vi "Ext.vi"(8 "error in (no error)":errorcluster, 9 "Val":variant, 10 "Tag":u16, 11 "Sine in":refnum<class "Rigol DG822 Sine.lvclass">) -> (0 "error out":errorcluster, 1 "Parsed":variant, 3 "Sine out":refnum<class "Rigol DG822 Sine.lvclass">)   [LabVIEW 2021, in "Rigol DG822 UI.lvlib" / "Rigol DG822 Sine.lvlib" / "Rigol DG822 Sine.lvclass"]
uses:
  Rigol DG822 Sine.lvclass
  Rigol DG822 UI/lib/controls.llb/WaveformExtCall.ctl
  Rigol DG822 Sine.lvclass/Rigol DG822 Sine.ctl
  Rigol DG822 UI/lib/controls.llb/AllWaveformDataCluster.ctl
  Rigol DG822 UI/lib/controls.llb/DataCluster.ctl
  Rigol DG822 UI/lib/controls.llb/FT Controls Cluster.ctl
  Rigol DG822 UI/lib/controls.llb/String Indicators Cluster.ctl
  General/Files/lvlibp/Actors.lvlibp/Actors/Actors/Actors.lvclass
  D:/LabVIEW/General/Files/lvlibp/Actors.lvlibp/Actors/Actors/Actors.lvclass
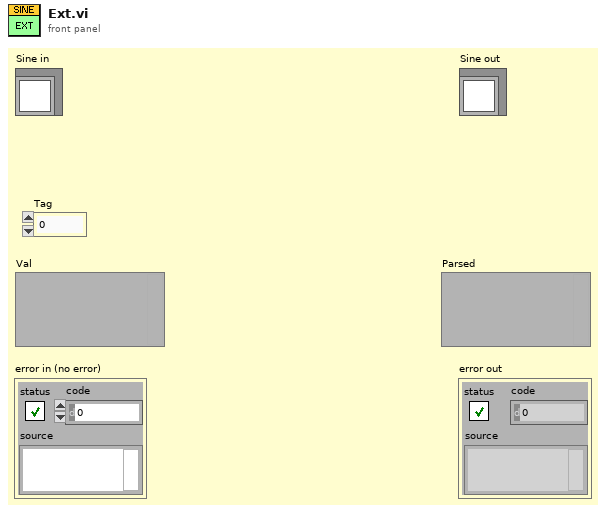
[diagram p1: front panel]
types:
  T1 = typedef "WaveformExtCall.ctl" = enum16{"Freq", "Period", "Ampl", "HighL", "Offset", "LowL", "Phase", "Duty", "Width", "RisEdge", "FallEdge", "Home", "InitData"}
  T2 = typedef "AllWaveformDataCluster.ctl" = cluster{"Data":T3, "F/T Ctrls":T4, "String Indcs":T5}
  T3 = typedef "DataCluster.ctl" = cluster{"Freq":cluster{"Freq":dbl, "FreqUnit":enum32{"No Selection", "MHz", "kHz", "Hz", "mHz", "uHz"}, "FreqUnitPrcs":dbl}, "Period":cluster{"Period":dbl, "PeriodUnit":enum32{"No Selection", "s", "ms", "us", "ns"}, "PeriodUnitPrcs":dbl}, "Ampl":cluster{"Ampl":dbl, "AmplUnit":enum32{"No Selection", "Vpp", "mVpp"}, "AmplUnitPrcs":dbl}, "HighL":cluster{"HighL":dbl, "HighLUnit":enum32{"No Selection", "V", "mV"}, "HighLUnitPrcs":dbl}, "Offset":cluster{"Offset":dbl, "OffsetUnit":enum32{"No Selection", "Vdc", "mVdc"}, "OffsetUnitPrcs":dbl}, "LowL":cluster{"LowL":dbl, "LowLUnit":enum32{"No Selection", "V", "mV"}, "LowLUnitPrcs":dbl}, "Phase":cluster{"Phase":dbl, "PhaseUnit":enum32{"°"}, "PhaseUnitPrcs":dbl}, "Duty":cluster{"Duty":dbl, "DutyUnit":enum32{"%"}, "DutyUnitPrcs":dbl}, "Width":cluster{"Width":dbl, "WidthUnit":enum32{"No Selection", "s", "ms", "us", "ns"}, "WidthUnitPrcs":dbl}, "RisEdge":cluster{"RisEdge":dbl, "RisEdgeUnit":enum32{"No Selection", "s", "ms", "us", "ns"}, "RisEdgeUnitPrcs":dbl}, "FallEdge":cluster{"FallEdge":dbl, "FallEdgeUnit":enum32{"No Selection", "s", "ms", "us", "ns"}, "FallEdgeUnitPrcs":dbl}}
  T4 = typedef "FT Controls Cluster.ctl" = cluster{"Freq/Period":bool, "Ampl/HighL":bool, "Offset/LowL":bool, "Duty/Width":bool}
  T5 = typedef "String Indicators Cluster.ctl" = cluster{"Freq-Period":string, "Ampl-HighL":string, "Offset-LowL":string, "Phase":string, "Duty-Width":string, "RisEdge":string, "FallEdge":string}
  T6 = cluster{"Freq":dbl, "FreqUnit":enum32{"No Selection", "MHz", "kHz", "Hz", "mHz", "uHz"}, "FreqUnitPrcs":dbl}
  T7 = cluster{"Period":dbl, "PeriodUnit":enum32{"No Selection", "s", "ms", "us", "ns"}, "PeriodUnitPrcs":dbl}
  T8 = cluster{"Freq":cluster{"Freq":dbl, "FreqUnit":enum32{"No Selection", "MHz", "kHz", "Hz", "mHz", "uHz"}, "FreqUnitPrcs":dbl}, "Period":cluster{"Period":dbl, "PeriodUnit":enum32{"No Selection", "s", "ms", "us", "ns"}, "PeriodUnitPrcs":dbl}}
  T9 = cluster{"Ampl":dbl, "AmplUnit":enum32{"No Selection", "Vpp", "mVpp"}, "AmplUnitPrcs":dbl}
  T10 = cluster{"HighL":dbl, "HighLUnit":enum32{"No Selection", "V", "mV"}, "HighLUnitPrcs":dbl}
  T11 = cluster{"Offset":dbl, "OffsetUnit":enum32{"No Selection", "Vdc", "mVdc"}, "OffsetUnitPrcs":dbl}
  T12 = cluster{"LowL":dbl, "LowLUnit":enum32{"No Selection", "V", "mV"}, "LowLUnitPrcs":dbl}
  T13 = cluster{"Ampl":cluster{"Ampl":dbl, "AmplUnit":enum32{"No Selection", "Vpp", "mVpp"}, "AmplUnitPrcs":dbl}, "HighL":cluster{"HighL":dbl, "HighLUnit":enum32{"No Selection", "V", "mV"}, "HighLUnitPrcs":dbl}, "Offset":cluster{"Offset":dbl, "OffsetUnit":enum32{"No Selection", "Vdc", "mVdc"}, "OffsetUnitPrcs":dbl}, "LowL":cluster{"LowL":dbl, "LowLUnit":enum32{"No Selection", "V", "mV"}, "LowLUnitPrcs":dbl}}
  T14 = cluster{"Phase":dbl, "PhaseUnit":enum32{"°"}, "PhaseUnitPrcs":dbl}
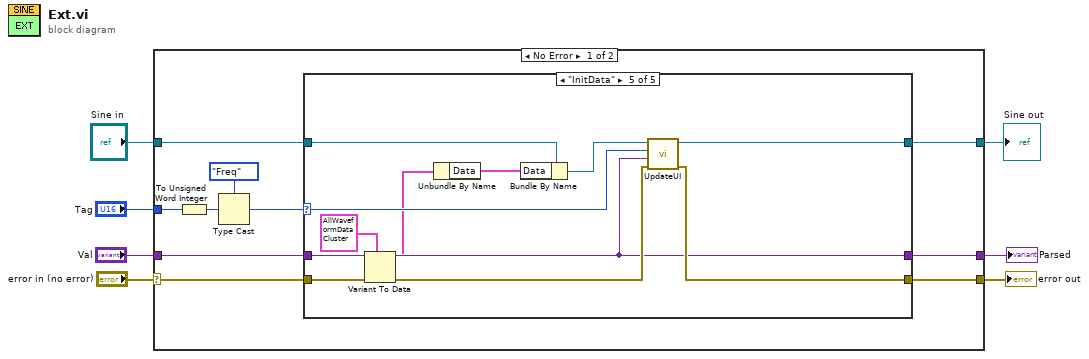
[diagram p0: block diagram]
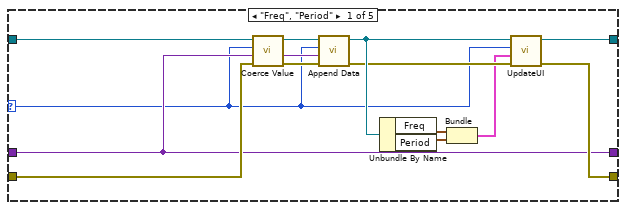
[diagram p2: hidden frame]
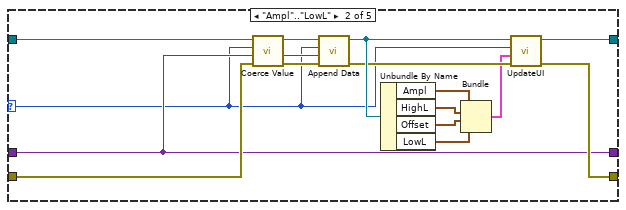
[diagram p3: hidden frame]
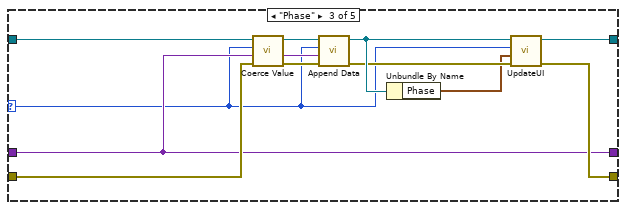
[diagram p4: hidden frame]
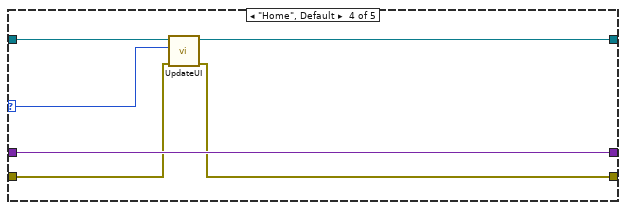
[diagram p5: hidden frame]
diagram:
  n1 = case shown="No Error" "error in (no error)" {
    selector: "error in (no error)" -> [w10 w78]
    tunnel: [w12 w77] -> w3
    tunnel: "Sine in" -> [w13 w77]
    tunnel: "Tag" -> [w16 _]
    tunnel: "Val" -> [w15 _]
    tunnel: [w11 _] -> w2
    tunnel: [w9 w78] -> w1
    frame No Error {
      n2 = To Unsigned Word Integer(number=w16) -> (unsigned 16bit integer=w17:u16)
      n3 = Type Cast(type=WaveformExtCall."Freq" ("Enum"), x=w17) -> (*(type *) &x=w14:T1)
      n4 = case shown="\"InitData\"" w14 {
        selector: w14 -> [w21 w37 w49 w63 w69]
        tunnel: w15 -> [w25 w41 w53 w62 w68]
        tunnel: w13 -> [w27 w43 w55 w65 w75]
        tunnel: [w31 w47 w59 w64 w76] -> w12
        tunnel: [w25 w41 w53 w62 w68] -> w11
        tunnel: w10 -> [w26 w42 w54 w61 w73]
        tunnel: [w30 w46 w58 w60 w70] -> w9
        frame "Freq", "Period" {
          n5 = call-dynamic "Coerce Value.vi"("error in (no error)"=w26, "Value"=w25, "ParamTags"=w21, "Rigol DG822 Sine in"=w27) -> ("error out"=w23:errorcluster, "Coerced Value"=w24:variant, "Rigol DG822 Sine out"=w28:refnum<class "Rigol DG822 Sine.lvclass">)  [unwired: 5 in]
          n6 = call-dynamic "Append Data.vi"("error in (no error)"=w23, "Data"=w24, "ParamTags"=w21, "Rigol DG822 Sine in"=w28) -> ("error out"=w22:errorcluster, "Rigol DG822 Sine out"=w29:refnum<class "Rigol DG822 Sine.lvclass">)  [unwired: 6 in]
          n7 = Unbundle By Name(w29) -> ("Freq"=w19:T6, "Period"=w18:T7)
          n8 = Bundle("Freq"=w19, "Period"=w18) -> (w20:T8)  [unwired: 1 in]
          n9 = call "UpdateUI.vi"("error in (no error)"=w22, "Data"=w20, "Type"=w21, "Recursive in"=w29) -> ("error out"=w30:errorcluster, "Recursive out"=w31:refnum<class "Rigol DG822 Sine.lvclass">)  [unwired: 6 in]
        }
        frame "Ampl".."LowL" {
          n10 = call-dynamic "Coerce Value.vi"("error in (no error)"=w42, "Value"=w41, "ParamTags"=w37, "Rigol DG822 Sine in"=w43) -> ("error out"=w39:errorcluster, "Coerced Value"=w40:variant, "Rigol DG822 Sine out"=w44:refnum<class "Rigol DG822 Sine.lvclass">)  [unwired: 5 in]
          n11 = call-dynamic "Append Data.vi"("error in (no error)"=w39, "Data"=w40, "ParamTags"=w37, "Rigol DG822 Sine in"=w44) -> ("error out"=w38:errorcluster, "Rigol DG822 Sine out"=w45:refnum<class "Rigol DG822 Sine.lvclass">)  [unwired: 6 in]
          n12 = Unbundle By Name(w45) -> ("Ampl"=w36:T9, "HighL"=w33:T10, "Offset"=w32:T11, "LowL"=w34:T12)
          n13 = Bundle("Ampl"=w36, "HighL"=w33, "Offset"=w32, "LowL"=w34) -> (w35:T13)  [unwired: 1 in]
          n14 = call "UpdateUI.vi"("error in (no error)"=w38, "Data"=w35, "Type"=w37, "Recursive in"=w45) -> ("error out"=w46:errorcluster, "Recursive out"=w47:refnum<class "Rigol DG822 Sine.lvclass">)  [unwired: 6 in]
        }
        frame "Phase" {
          n15 = call-dynamic "Coerce Value.vi"("error in (no error)"=w54, "Value"=w53, "ParamTags"=w49, "Rigol DG822 Sine in"=w55) -> ("error out"=w51:errorcluster, "Coerced Value"=w52:variant, "Rigol DG822 Sine out"=w56:refnum<class "Rigol DG822 Sine.lvclass">)  [unwired: 5 in]
          n16 = call-dynamic "Append Data.vi"("error in (no error)"=w51, "Data"=w52, "ParamTags"=w49, "Rigol DG822 Sine in"=w56) -> ("error out"=w50:errorcluster, "Rigol DG822 Sine out"=w57:refnum<class "Rigol DG822 Sine.lvclass">)  [unwired: 6 in]
          n17 = Unbundle By Name(w57) -> ("Phase"=w48:T14)
          n18 = call "UpdateUI.vi"("error in (no error)"=w50, "Data"=w48, "Type"=w49, "Recursive in"=w57) -> ("error out"=w58:errorcluster, "Recursive out"=w59:refnum<class "Rigol DG822 Sine.lvclass">)  [unwired: 6 in]
        }
        frame "Home", Default {
          n19 = call "UpdateUI.vi"("error in (no error)"=w61, "Type"=w63, "Recursive in"=w65) -> ("error out"=w60:errorcluster, "Recursive out"=w64:refnum<class "Rigol DG822 Sine.lvclass">)  [unwired: 7 in]
        }
        frame "InitData" {
          n20 = Variant To Data(error in=w73, type=T2 {"Data"={"Freq"={"Freq"=1.0, "FreqUnit"=enum."kHz", "FreqUnitPrcs"=9.0}, "Period"={"Period"=1.0, "PeriodUnit"=enum."ms", "PeriodUnitPrcs"=7.0}, "Ampl"={"Ampl"=5.0, "AmplUnit"=enum."Vpp", "AmplUnitPrcs"=4.0}, "HighL"={"HighL"=2.5, "HighLUnit"=enum."V", "HighLUnitPrcs"=4.0}, "Offset"={"Offset"=0.0, "OffsetUnit"=enum."Vdc", "OffsetUnitPrcs"=4.0}, "LowL"={"LowL"=-2.5, "LowLUnit"=enum."V", "LowLUnitPrcs"=4.0}, "Phase"={"Phase"=0.0, "PhaseUnit"=enum."°", "PhaseUnitPrcs"=3.0}, "Duty"={"Duty"=50.0, "DutyUnit"=enum."%", "DutyUnitPrcs"=3.0}, "Width"={"Width"=500.0, "WidthUnit"=enum."us", "WidthUnitPrcs"=4.0}, "RisEdge"={"RisEdge"=10.0, "RisEdgeUnit"=enum."ns", "RisEdgeUnitPrcs"=1.0}, "FallEdge"={"FallEdge"=10.0, "FallEdgeUnit"=enum."ns", "FallEdgeUnitPrcs"=1.0}}, "F/T Ctrls"={"Freq/Period"=FALSE, "Ampl/HighL"=FALSE, "Offset/LowL"=FALSE, "Duty/Width"=FALSE}, "String Indcs"={"Freq-Period"="1.000,000,000 kHz", "Ampl-HighL"="5.000,0 Vpp", "Offset-LowL"="0.000,0 Vdc", "Phase"="0.000 °", "Duty-Width"="50.000 %", "RisEdge"="10.0 ns", "FallEdge"="10.0 ns"}} ("Params Data"), Variant=w68) -> (data=w67:T2, error out=w72:errorcluster)
          n21 = Unbundle By Name(w67) -> ("Data"=w71:T3)
          n22 = Bundle By Name(cluster=w75, "Data"=w71) -> (w74:refnum<class "Rigol DG822 Sine.lvclass">)
          n23 = call "UpdateUI.vi"("error in (no error)"=w72, "Data"=w68, "Type"=w69, "Recursive in"=w74) -> ("error out"=w70:errorcluster, "Recursive out"=w76:refnum<class "Rigol DG822 Sine.lvclass">)  [unwired: 6 in]
        }
      }
    }
    frame Error {
    }
  }
  "error out" <- w1
  "Sine out" <- w3
  "Parsed" <- w2
